vi "RawUnitsToRPM.vi"   [LabVIEW 2020, in "TitanLib.lvlib"]
uses:
  TitanLib.lvlib
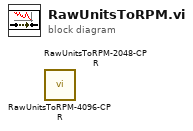
[diagram p0: block diagram]
diagram:
  n1 = call "RawUnitsToRPM-4096-CPR.vi"() -> ()  [unwired: 4 in, 1 out]
  n2 = call "RawUnitsToRPM-2048-CPR.vi"() -> ()  [unwired: 4 in, 1 out]
